vi "TestPc.vi"() -> ()   [LabVIEW 2017]
panel:
  in  "Slide 2":dbl(slide) scale=0.0..10.0
  in  "Slide":dbl(slide) scale=0.0..10.0
  in  "stop":bool
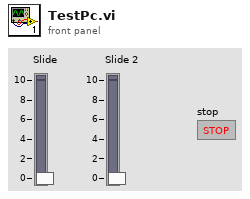
[diagram p1: front panel]
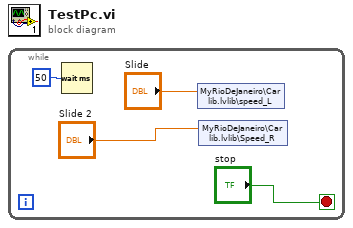
[diagram p0: block diagram]
diagram:
  n1 = while {
    stop <- "stop" stop-if-true
    n2 = Wait (ms)(milliseconds to wait=u32 50) -> ()  [unwired: 1 out]
    n3 = shared-variable "MyRioDeJaneiro\\Car lib.lvlib\\speed_L"("Slide") -> ()  [unwired: 1 in, 1 out]
    n4 = shared-variable "MyRioDeJaneiro\\Car lib.lvlib\\Speed_R"("Slide 2") -> ()  [unwired: 1 in, 1 out]
  }
